vi "Supply_ComplianceCheck.vi"(8 "error in (no error)":errorcluster, 11 "KE236 in":refnum<class "KE236.lvclass">) -> (0 "error out":errorcluster, 1 "Status string":string, 2 "Compliance exceeded?":bool, 3 "KE236 out":refnum<class "KE236.lvclass">)   [LabVIEW 2013, in "KE236.lvclass"]
uses:
  KE236.lvclass
  SupplyControl.lvclass
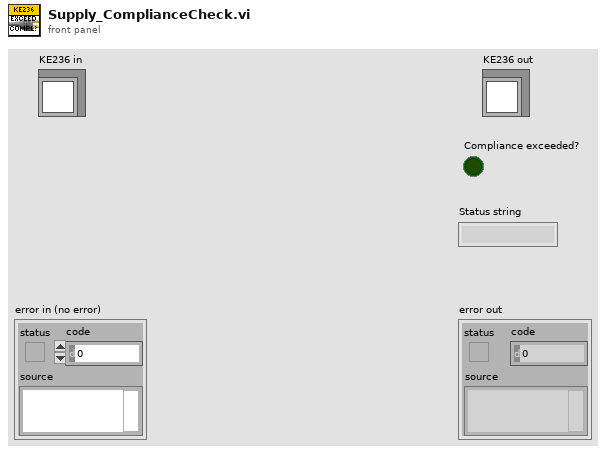
[diagram p1: front panel]
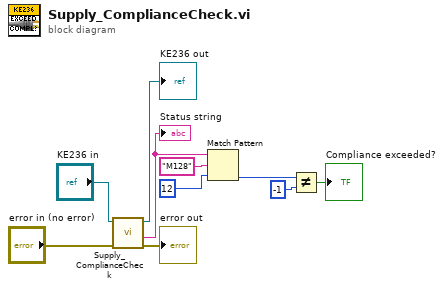
[diagram p0: block diagram]
diagram:
  n1 = call-parent "Supply_ComplianceCheck.vi"("error in (no error)"="error in (no error)", "SupplyControl in"="KE236 in") -> ("error out"=→"error out":errorcluster, "Status string"=w2:string, "SupplyControl out"=→"KE236 out":refnum<class "KE236.lvclass">)  [unwired: 6 in, 1 out]
  "Status string" <- w2
  n2 = Match Pattern(string=w2, regular expression="M128", offset (0)=12) -> (offset past match=w5:i32)  [unwired: 3 out]
  n3 = Not Equal?(x=w5, y=-1) -> (x != y?=→"Compliance exceeded?":bool)
